vi "Read Charact Standard List.vi"(8 "error in":errorcluster, 11 "SG Path Group in":refnum<class "SG Path Group.lvclass">) -> (0 "error out":errorcluster, 2 "Charact Standard List":T1[](array[typedef]), 3 "SG Path Group out":refnum<class "SG Path Group.lvclass">)   [LabVIEW 2023, in "RFFixtureCharact.RMM.lvlib" / "SG Path Group.lvclass"]
uses:
  SG Path Group.lvclass
  Instruments/Cal Standard/Type Definitions/Standard Type.ctl
  SG Path Group.lvclass/SG Path Group.ctl
  Instruments/RFFixtureCharact.Instruments.lvlib
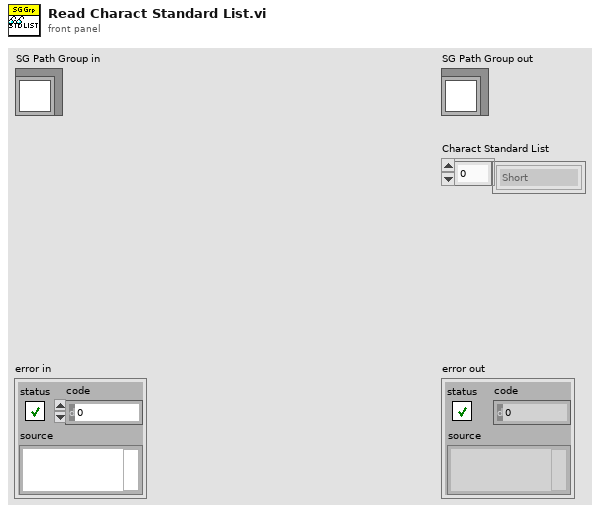
[diagram p1: front panel]
types:
  T1 = typedef "RFFixtureCharact.Instruments.lvlib/Standard Type.ctl" = enum16{"Short", "Open", "Load", "PowerMeter", "None"}
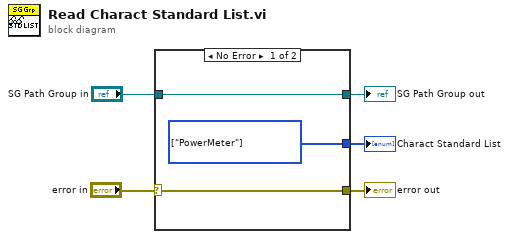
[diagram p0: block diagram]
diagram:
  n1 = case shown="No Error" "error in" {
    selector: "error in" -> [w6 w9]
    tunnel: [w8 _] -> w5
    tunnel: [w7 w10] -> w4
    tunnel: "SG Path Group in" -> [w7 w10]
    tunnel: [w6 w9] -> w1
    frame No Error {
      w8 = T1[] [enum."PowerMeter"] items=["Short", "Open", "Load", "PowerMeter", "None"] ("Charact Standard List")
    }
    frame Error {
    }
  }
  "error out" <- w1
  "SG Path Group out" <- w4
  "Charact Standard List" <- w5
